vi "LINX - UART Loopback Benchmark.vi"() -> ()   [LabVIEW 2019]
uses:
  <vilib>/MakerHub/LINX/Public/Peripherals/UART/UART Write String.vi
  <vilib>/MakerHub/LINX/Public/Peripherals/UART/UART Write Byte Array.vi
  <vilib>/MakerHub/LINX/Private/Local IO/LinxUartWrite.vi
  <vilib>/MakerHub/LINX/Public/Utilities/Check Channel.vi
  <vilib>/MakerHub/LINX/Public/Utilities/Open Local.vi
  <vilib>/MakerHub/LINX/Private/Utilties/Generate Error.vi
  <vilib>/MakerHub/LINX/Public/Peripherals/UART/UART Read String.vi
  <vilib>/MakerHub/LINX/LMH-LINX.lvlib
panel:
  out "Read Data":string
  in  "Write Data":string
  out "Actual Baud":u32
  in  "Baud Rate":u32=9600
  in  "Warmup Iterations":i32=100
  out "Chart":dbl(graph)
  in  "Stop Button":bool
  in  "Benchmark Iterations":i32=1000
  out "Samples Per Second":i32
  in  "UART Channel":u8=7
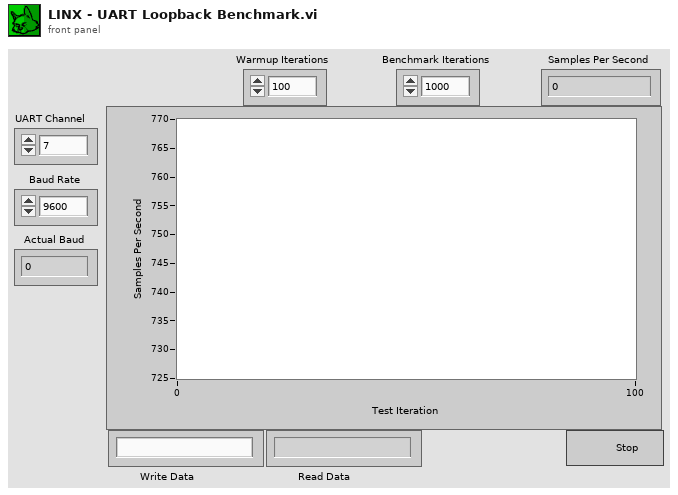
[diagram p1: front panel]
types:
  T1 = typedef "LMH-LINX.lvlib/LINX Ref.ctl" = cluster{"IO":T2, "Interface":T3, "LINX Device Config":T4}
  T2 = typedef "LMH-LINX.lvlib/Platform.ctl" = enum16{"Remote", "Local"}
  T3 = typedef "LMH-LINX.lvlib/Interface.ctl" = enum16{"Serial", "TCP"}
  T4 = typedef "LMH-LINX.lvlib/Device.lvlib/LINX Device Config.ctl" = cluster{"Interface":T3, "COM Port":refnum<visa-resource-name>, "TCP Configuration":T5, "Device Family":u8, "Device ID":u8, "Device Name":string, "TCP Ref":refnum<k5>, "Channels":T6}
  T5 = typedef "LMH-LINX.lvlib/Device.lvlib/TCP Config.ctl" = cluster{"IP Address":string, "Port":u16}
  T6 = typedef "LMH-LINX.lvlib/Channels.ctl" = cluster{"DI":u8[], "DO":u8[], "AI":u8[], "AO":u8[], "PWM":u8[], "QE":u8[], "UART":u8[], "I2C 2":u8[], "SPI":u8[], "CAN":u8[], "Servo":u8[], "AI Ref (V)":dbl, "AI Resolution (Bits)":u8, "AO Ref (V)":dbl, "AO Resolution (Bits)":u8}
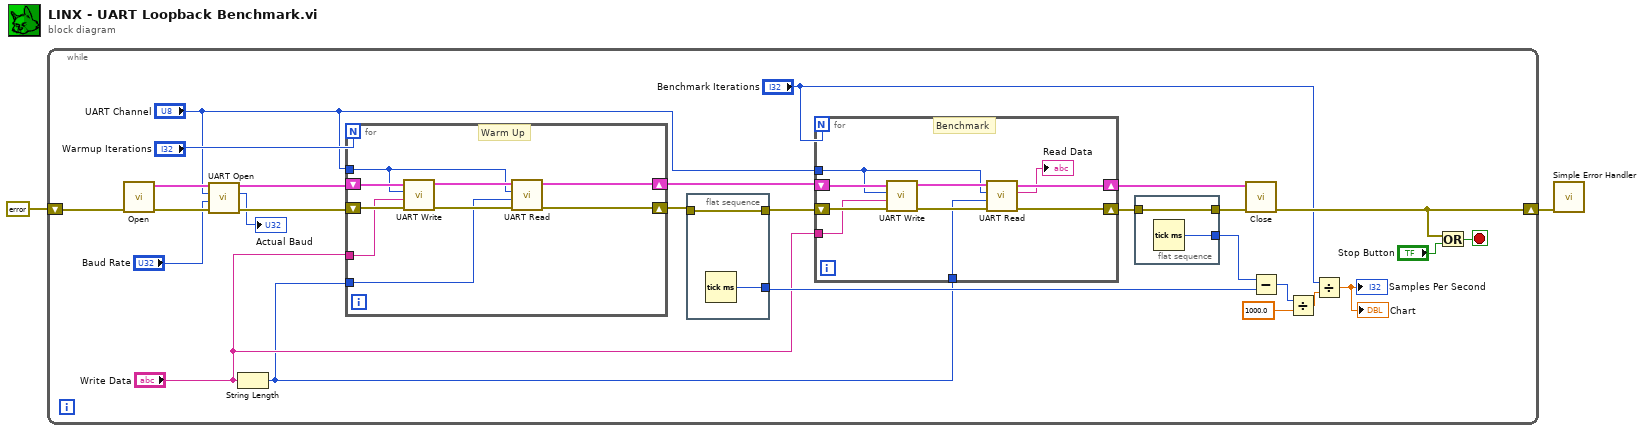
[diagram p0: block diagram]
diagram:
  n1 = while {
    shift-right: [w22] -> w2
    shift-left: errorcluster {"status"=FALSE, "code"=0, "source"=""} ("Error Out") -> [w20]
    stop <- w12 stop-if-true
    n2 = call-poly <vilib>:"Open.vi"("Error In"=w20) -> ("Error Out"=w11:errorcluster, "LINX Resource"=w10:T1)  [unwired: 8 in, 1 out]
    n3 = call <vilib>:"UART Open.vi"("Error In"=w11, "Baud Rate (9600)"="Baud Rate", "UART Channel (0)"="UART Channel", "LINX Resource"=w10) -> ("Error Out"=w9:errorcluster, "Actual Baud"=→"Actual Baud":u32, "LINX Resource"=w8:T1)  [unwired: 5 in]
    n4 = String Length(string="Write Data") -> (length=w3:i32)
    n5 = for {
      N: "Warmup Iterations" -> [_]
      shift-right: [w35] -> w24
      shift-left: w8 -> [w38]
      shift-right: [w34] -> w25
      shift-left: w9 -> [w37]
      tunnel: "UART Channel" -> [w32]
      tunnel: "Write Data" -> [w31]
      tunnel: w3 -> [w30]
      # "Warm Up"
      n6 = call-poly <vilib>:"UART Write.vi"("Error In"=w37, "Data"=w31, "UART Channel (0)"=w32, "LINX Resource"=w38) -> ("Error Out"=w33:errorcluster, "LINX Resource"=w36:T1)  [unwired: 6 in]
      n7 = call-poly <vilib>:"UART Read.vi"("Error In"=w33, "Num Bytes"=w30, "UART Channel (0)"=w32, "LINX Resource"=w36) -> ("Error Out"=w34:errorcluster, "LINX Resource"=w35:T1)  [unwired: 5 in, 1 out]
    }
    n8 = flat-sequence {
      tunnel: [w52] -> w28
      tunnel: w25 -> [w52]
      tunnel: [w51] -> w15
      frame #0 {
        n9 = Tick Count (ms)() -> (millisecond timer value=w51:u32)
      }
    }
    n10 = for {
      N: "Benchmark Iterations" -> [_]
      shift-right: [w45] -> w29
      shift-left: w24 -> [w47]
      shift-right: [w44] -> w27
      shift-left: w28 -> [w43]
      tunnel: "UART Channel" -> [w40]
      tunnel: "Write Data" -> [w42]
      tunnel: w3 -> [w41]
      # "Benchmark"
      n11 = call-poly <vilib>:"UART Write.vi"("Error In"=w43, "Data"=w42, "UART Channel (0)"=w40, "LINX Resource"=w47) -> ("Error Out"=w48:errorcluster, "LINX Resource"=w46:T1)  [unwired: 6 in]
      n12 = call-poly <vilib>:"UART Read.vi"("Error In"=w48, "Num Bytes"=w41, "UART Channel (0)"=w40, "LINX Resource"=w46) -> ("Error Out"=w44:errorcluster, "Data"=→"Read Data":string, "LINX Resource"=w45:T1)  [unwired: 5 in]
    }
    n13 = flat-sequence {
      tunnel: [w50] -> w26
      tunnel: w27 -> [w50]
      tunnel: [w49] -> w16
      frame #0 {
        n14 = Tick Count (ms)() -> (millisecond timer value=w49:u32)
      }
    }
    n15 = call <vilib>:"Close.vi"("Error In"=w26, "LINX Resource"=w29) -> ("Error Out"=w22:errorcluster)  [unwired: 9 in]
    n16 = Subtract(x=w16, y=w15) -> (x-y=w19:u32)
    n17 = Divide(x=w19, y=1000.0) -> (x/y=w18:dbl)
    n18 = Divide(x="Benchmark Iterations", y=w18) -> (x/y=→"Chart" →"Samples Per Second":dbl)
    n19 = Or(x=w22, y="Stop Button") -> (x .or. y?=w12:bool)
  }
  n20 = call <vilib>:"Simple Error Handler.vi"("error in (no error)"=w2) -> ()  [unwired: 4 in, 5 out]
